vi "Feed.vi"() -> ()   [LabVIEW 2014]
uses:
  subVI/version.vi
panel:
  in  "닫기":bool
  in  "전송":bool
  in  "Message":string caption="메시지"
  # "개발자에게 피드백"
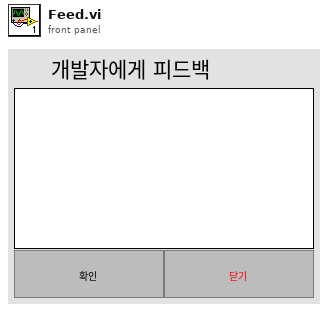
[diagram p1: front panel]
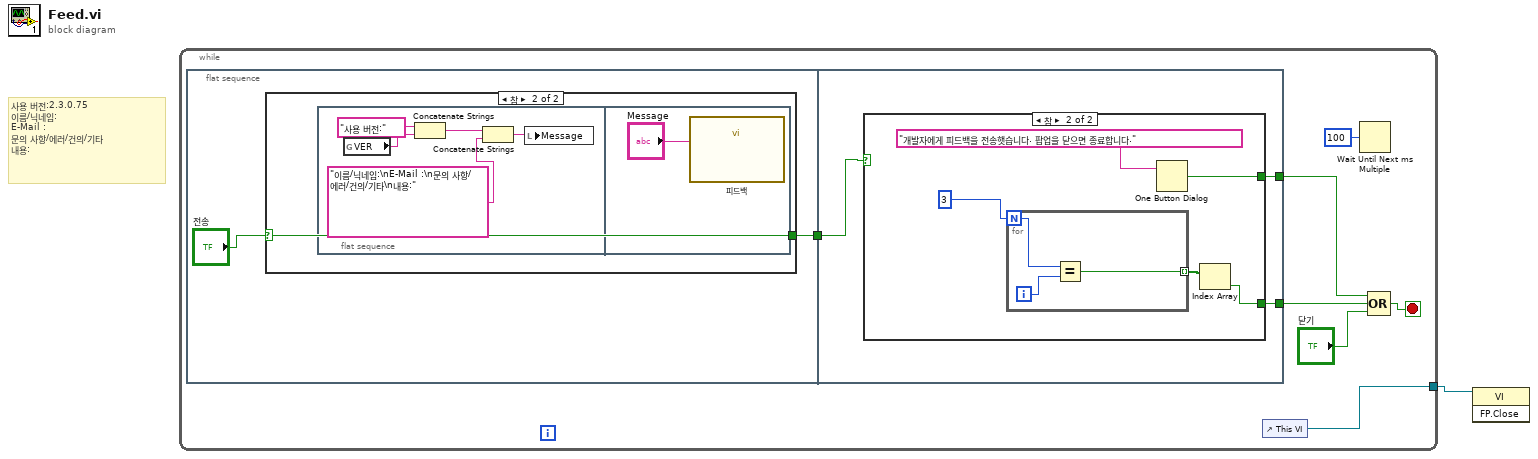
[diagram p0: block diagram]
diagram:
  # "사용 버전:2.3.0.75\n이름/닉네임:\nE-Mail :\n문의 사항/에러/건의/기타\n내용:"
  n1 = while {
    tunnel: [w8] -> w1
    stop <- w3 stop-if-true
    n2 = flat-sequence {
      tunnel: [w9] -> w7
      tunnel: w7 -> [w20]
      tunnel: [w19] -> w4
      tunnel: [w18] -> w5
      frame #0 {
        n3 = case shown="참" "전송" {
          selector: "전송" -> [_ w11]
          tunnel: [_ w11] -> w9
          frame False {
          }
          frame True {
            n4 = flat-sequence {
              frame #0 {
                n5 = global read "version.vi" "VER"() -> (w12:string)
                n6 = Concatenate Strings("사용 버전:" ("문자열"), w12) -> (w14:string)
                n7 = Concatenate Strings(w14, "이름/닉네임:\nE-Mail :\n문의 사항/에러/건의/기타\n내용:" ("문자열")) -> (w16:string)
                n8 = local write "Message"(w16) -> ()
              }
              frame #1 {
                n9 = call "피드백"("Message"="Message") -> ()  [unwired: 10 in, 1 out]
              }
            }
          }
        }
      }
      frame #1 {
        n10 = case shown="참" w20 {
          tunnel: [_ w24] -> w19
          tunnel: [_ w21] -> w18
          frame False {
          }
          frame True {
            n11 = for {
              N: 3 -> [w27]
              tunnel: [w26] -> w22 mode=indexing
              i -> [w28]
              n12 = Equal?(x=w27, y=w28) -> (x = y?=w26:bool)
            }
            n13 = One Button Dialog(message="개발자에게 피드백을 전송햇습니다. 팝업을 닫으면 종료합니다." ("메시지")) -> (true=w24:bool)  [unwired: 1 in]
            n14 = Index Array(array=w22) -> (element=w21:bool)  [unwired: 1 in]
          }
        }
      }
    }
    n15 = control-ref of="This VI"() -> (w8:refnum<vi>)
    n16 = Wait Until Next ms Multiple(millisecond multiple=u32 100 ("ms 배수")) -> ()  [unwired: 1 out]
    n17 = Compound Arithmetic op=OR(w4, w5, "닫기") -> (w3:bool)
  }
  n18 = invoke class="VI" method="FP.Close"(reference=w1) -> ()  [unwired: 2 in, 3 out]
